vi "Teleop Drive Dispatch.vi"(10 "array":dbl[](array[numeric])) -> ()   [LabVIEW 2017]
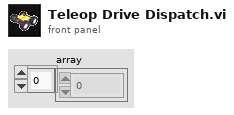
[diagram p1: front panel]
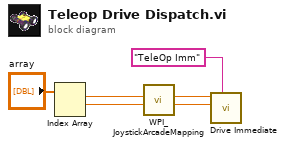
[diagram p0: block diagram]
diagram:
  n1 = Index Array(array="array") -> (element #1=w3:dbl, element #2=w2:dbl)  [unwired: 2 in]
  n2 = call <vilib>:"WPI_JoystickArcadeMapping.vi"("Y axis value"=w2, "X axis value"=w3) -> ("Right Motor Value"=w4:dbl, "Left Motor Value"=w5:dbl)  [unwired: 8 in]
  n3 = call "Drive Immediate.vi"("Description"="TeleOp Imm", "Right Setpoint"=w4, "Left Setpoint"=w5) -> ()  [unwired: 8 in, 1 out]
